vi "Online_Program_redesign_For_TV.vi"() -> ()   [LabVIEW 2014]
uses:
  <vilib>/Utility/file.llb/Read From Spreadsheet File (DBL).vi
  <vilib>/Analysis/Matrix/Numeric/Conversions/Array To Matrix - RA2.vi
  <vilib>/Instr/_visa.llb/VISA Configure Serial Port (Instr).vi
  <vilib>/Analysis/Matrix/Numeric/Conversions/Array To Matrix - RA.vi
  <vilib>/Utility/file.llb/Write To Spreadsheet File (DBL).vi
  <vilib>/Utility/file.llb/Write To Spreadsheet File (I64).vi
  <vilib>/Analysis/Matrix/NI_Matrix.lvlib
  NeuroSky_Dll_Call/Debug/NeuroSky_Dll_Call.dll
  user32.dll
panel:
  out "에러 출력":errorcluster
  out "메시지 2":string
  out "큐사인":bool
  out "icon_온도":bool
  out "icon_용변":bool
  out "icon_자판":bool
  out "icon_응급":bool=TRUE
  out "icon_기계":bool
  out "icon_침대":bool
  out "메시지":string
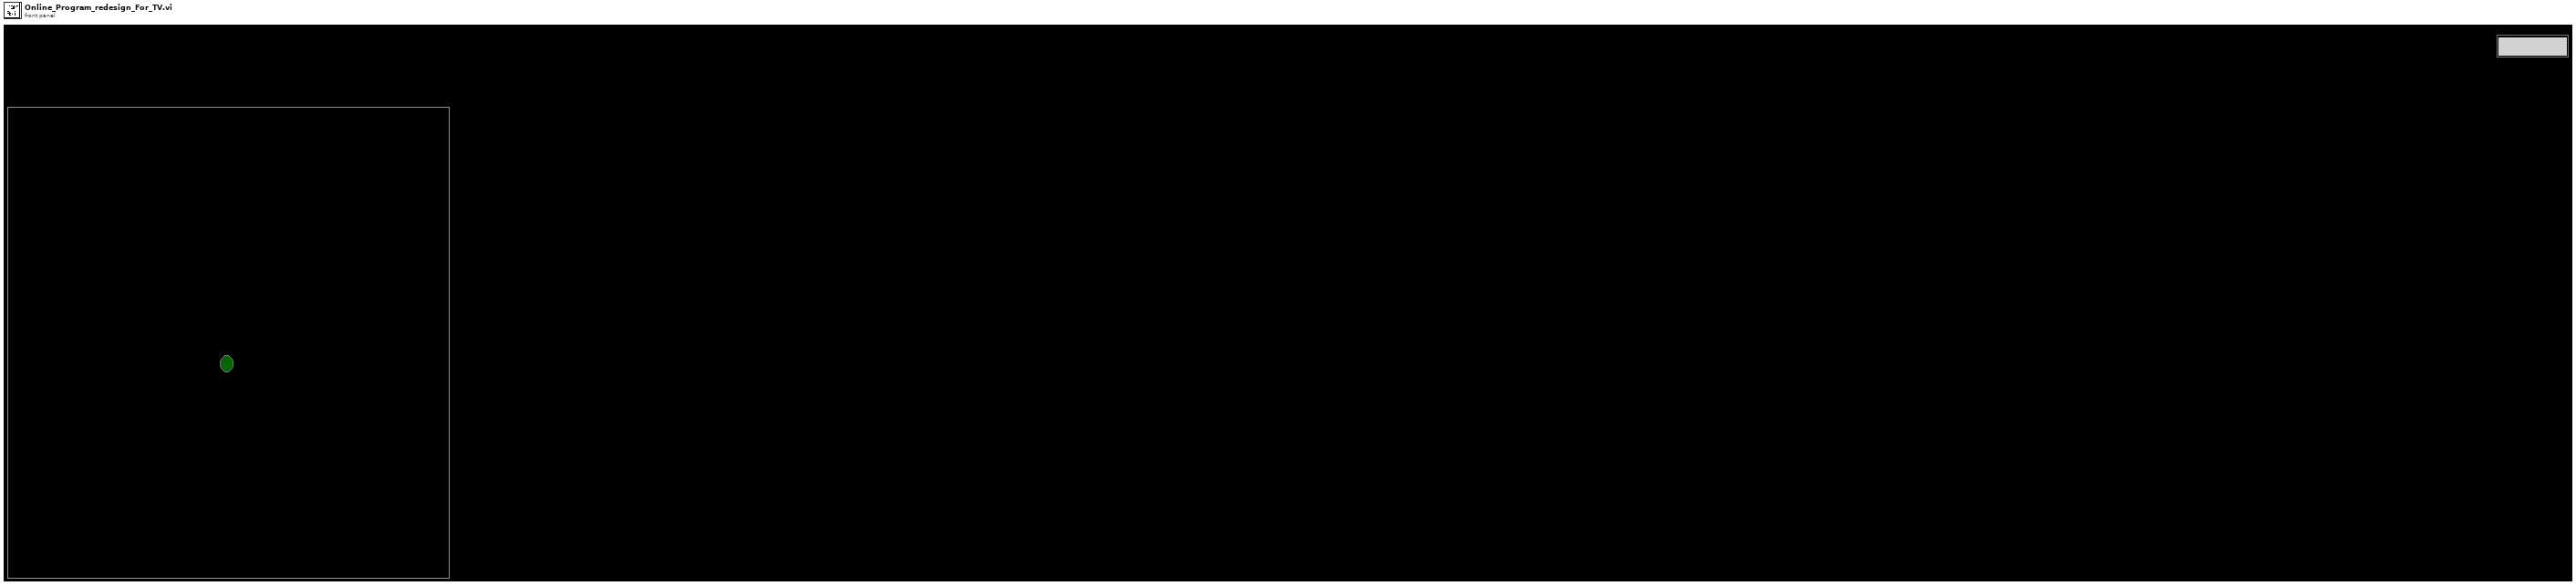
[diagram p1: front panel]
types:
  T1 = typedef "NI_Matrix.lvlib/RealMatrix.ctl" = dbl[][]
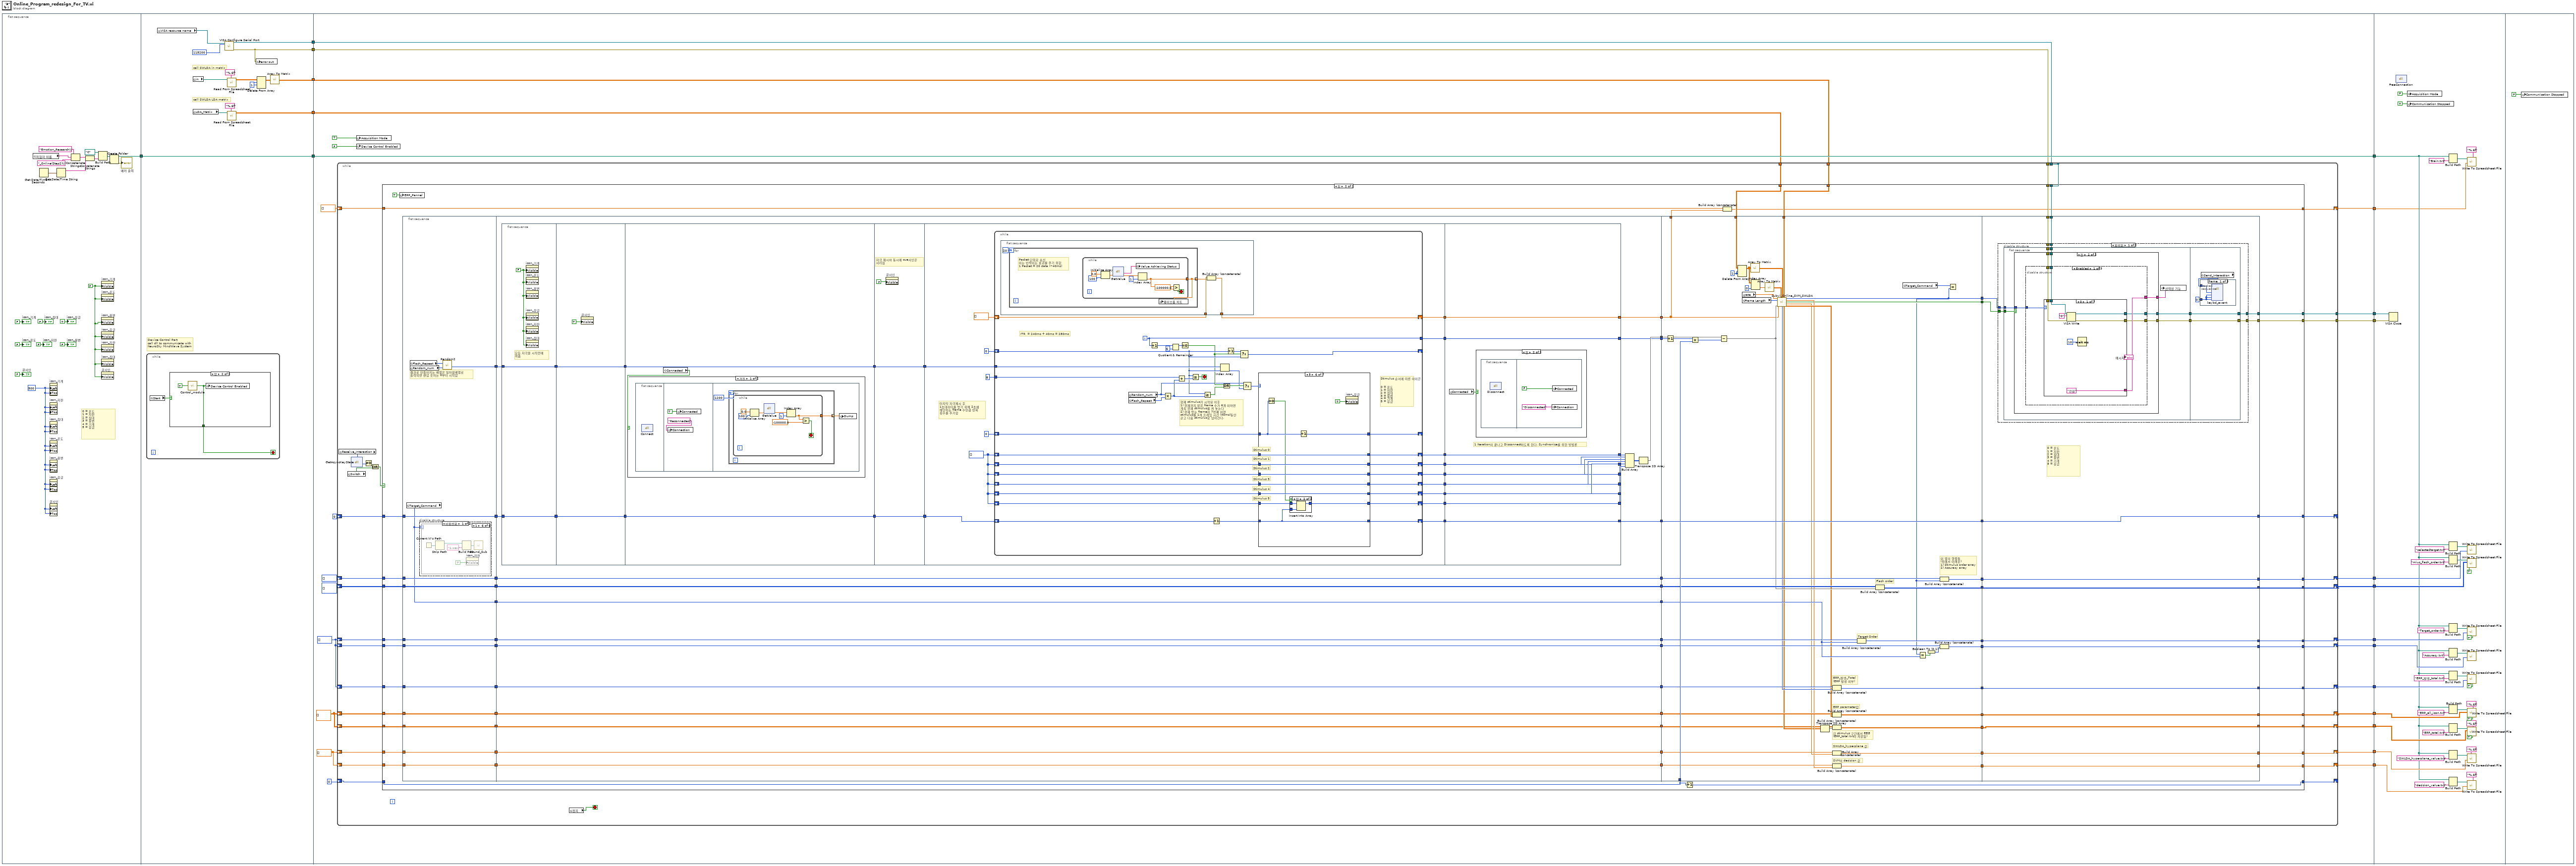
[diagram p0: block diagram]
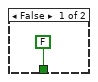
[diagram p2: hidden frame]
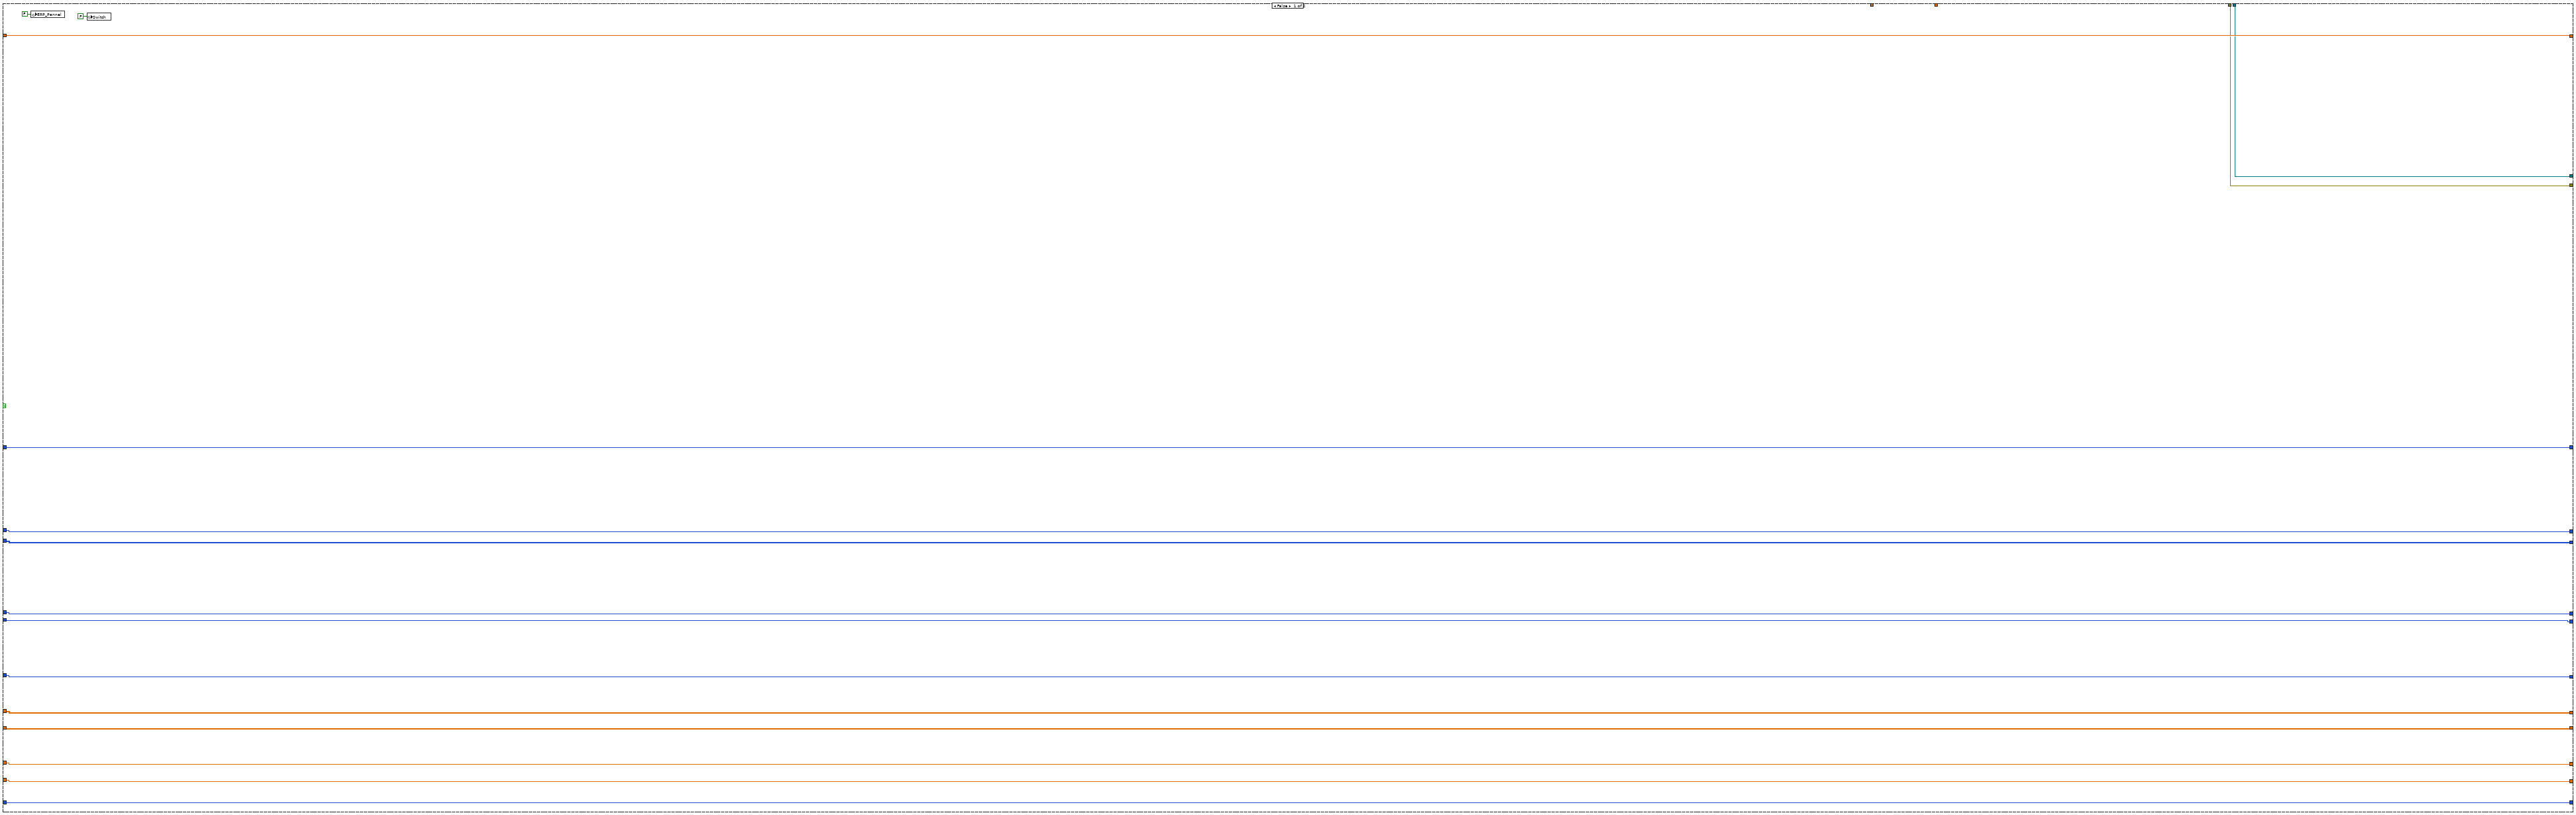
[diagram p3: hidden frame]
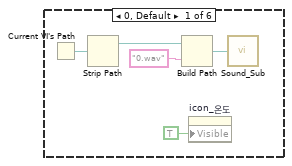
[diagram p4: hidden frame]
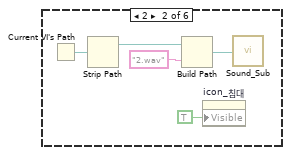
[diagram p5: hidden frame]
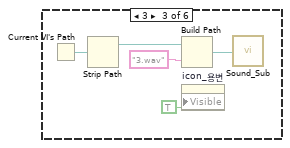
[diagram p6: hidden frame]
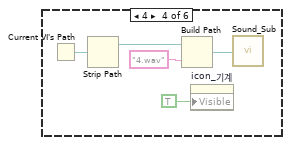
[diagram p7: hidden frame]
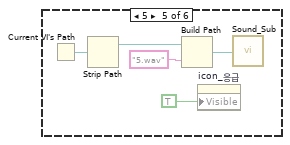
[diagram p8: hidden frame]
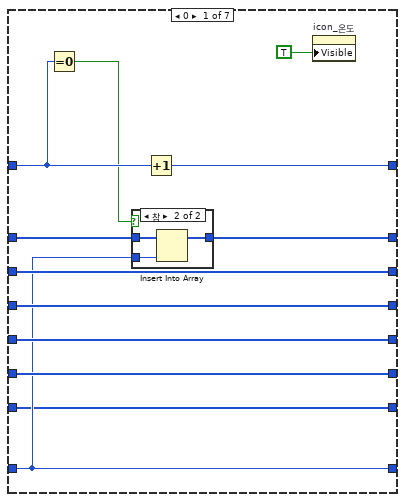
[diagram p11: hidden frame]
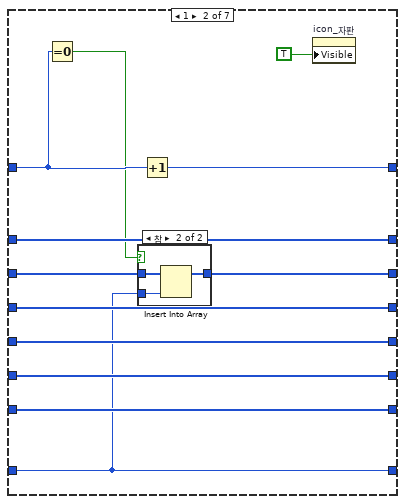
[diagram p13: hidden frame]
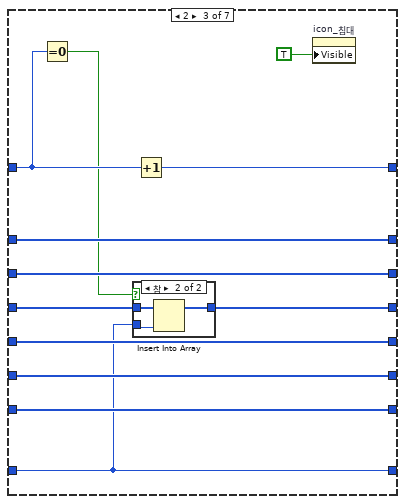
[diagram p15: hidden frame]
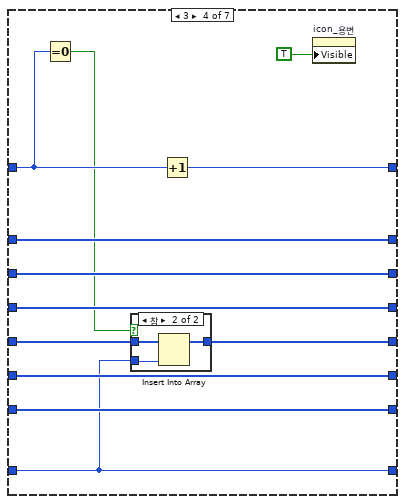
[diagram p17: hidden frame]
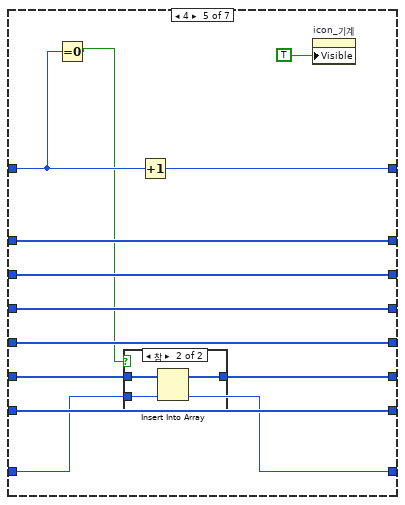
[diagram p19: hidden frame]
diagram:
  n1 = flat-sequence {
    tunnel: [w39] -> w19
    tunnel: w19 -> [w53]
    tunnel: [w53] -> w18
    tunnel: [w51] -> w17
    tunnel: [w44] -> w7
    tunnel: [w43] -> w4
    tunnel: [w40] -> w3
    tunnel: w18 -> [w76]
    tunnel: [w76] -> w16
    tunnel: [w85] -> w15
    tunnel: [w83] -> w14
    tunnel: [w81] -> w13
    tunnel: w17 -> [w65]
    tunnel: [w80] -> w12
    tunnel: [w77] -> w11
    tunnel: [w73] -> w10
    tunnel: [w71] -> w9
    tunnel: [w70] -> w8
    tunnel: w7 -> [w64]
    tunnel: [w68] -> w6
    tunnel: [w66] -> w5
    tunnel: w4 -> [w63]
    tunnel: w3 -> [w62]
    tunnel: [w61] -> w2
    tunnel: [w60] -> w1
    tunnel: w16 -> [w723]
    tunnel: w15 -> [w718]
    tunnel: w14 -> [w757]
    tunnel: w13 -> [w753]
    tunnel: w12 -> [w750]
    tunnel: w11 -> [w746]
    tunnel: w10 -> [w740]
    tunnel: w9 -> [w735]
    tunnel: w8 -> [w732]
    tunnel: w6 -> [w729]
    tunnel: w5 -> [w724]
    tunnel: w2 -> [w720]
    tunnel: w1 -> [w719]
    frame #0 {
      w20 = FALSE ("Visible")
      w22 = 500 ("Position:Left")
      # "0 = 온도\n1 = 자판\n2 = 침대\n3 = 용변 \n4 = 기계 \n5 = 응급"
      n2 = global read "Control_Panel_정리.vi" "피험자 이름"() -> (w30:string)
      n3 = Get Date/Time In Seconds() -> (seconds since 1Jan1904=w36:timestamp)
      n4 = property on="icon_기계" class="Bool (엄격한)"("Left"=w22, "Top"=w22) -> ()  [unwired: 2 in, 2 out]
      n5 = property on="icon_자판" class="Bool (엄격한)"("Left"=w22, "Top"=w22) -> ()  [unwired: 2 in, 2 out]
      n6 = property on="icon_침대" class="Bool (엄격한)"("Left"=w22, "Top"=w22) -> ()  [unwired: 2 in, 2 out]
      n7 = property on="icon_온도" class="Bool (엄격한)"("Left"=w22, "Top"=w22) -> ()  [unwired: 2 in, 2 out]
      n8 = property on="icon_용변" class="Bool (엄격한)"("Left"=w22, "Top"=w22) -> ()  [unwired: 2 in, 2 out]
      n9 = property on="icon_응급" class="Bool (엄격한)"("Left"=w22, "Top"=w22) -> ()  [unwired: 2 in, 2 out]
      n10 = property on="큐사인" class="Bool (엄격한)"("Left"=w22, "Top"=w22) -> ()  [unwired: 2 in, 2 out]
      n11 = Get Date/Time String(seconds (now)=w36) -> (date string=w37:string)  [unwired: 2 in, 1 out]
      n12 = Concatenate Strings("Emotion_Research\\" ("string"), w30, "_Online(Step2)\\" ("문자열")) -> (w32:string)
      n13 = Concatenate Strings(w32, w37) -> (w34:string)
      n14 = Build Path(base path=path "C:/" ("path"), name or relative path=w34) -> (appended path=w35:path)
      n15 = property on="icon_기계" class="Bool (엄격한)"("Visible"=w20) -> ()  [unwired: 2 in, 2 out]
      n16 = property on="icon_온도" class="Bool (엄격한)"("Visible"=w20) -> ()  [unwired: 2 in, 2 out]
      n17 = property on="icon_용변" class="Bool (엄격한)"("Visible"=w20) -> ()  [unwired: 2 in, 2 out]
      n18 = property on="icon_응급" class="Bool (엄격한)"("Visible"=w20) -> ()  [unwired: 2 in, 2 out]
      n19 = property on="icon_자판" class="Bool (엄격한)"("Visible"=w20) -> ()  [unwired: 2 in, 2 out]
      n20 = property on="icon_침대" class="Bool (엄격한)"("Visible"=w20) -> ()  [unwired: 2 in, 2 out]
      n21 = property on="큐사인" class="Bool (엄격한)"("Visible"=w20) -> ()  [unwired: 2 in, 2 out]
      n22 = Create Folder(path (use dialog)=w35) -> (created path=w39:path, error out=→"에러 출력":errorcluster)  [unwired: 2 in, 1 out]
      "icon_온도" <- FALSE ("icon_전원 6")
      "icon_용변" <- FALSE ("icon_전체종료")
      "icon_자판" <- FALSE ("icon_음량업 2")
      "icon_응급" <- TRUE ("icon_채널다운")
      "icon_기계" <- FALSE ("icon_음량다")
      "icon_침대" <- FALSE ("icon_채널업")
      "큐사인" <- FALSE ("icon_전원 7")
    }
    frame #1 {
      w47 = 1 ("인덱스 (행)")
      # "call SWLDA in matrix"
      # "call SWLDA LDA matrix"
      # "Device Control Part\ncall dll to communicate with\nNeuroSky MindWave System"
      n23 = while {
        stop <- w55 stop-if-true
        n24 = global read "Control_Panel_정리.vi" "Start"() -> (w54:bool)
        n25 = case shown="참" w54 {
          tunnel: [FALSE ("Connected") w57] -> w55
          frame False {
          }
          frame True {
            n26 = call "Control_module.vi"("Turn on"=TRUE ("Device Control Enabled")) -> ("Connected"=w57:bool)
            n27 = global write "Control_Panel_정리.vi" "Device Control Enabled"(w57) -> ()
          }
        }
      }
      n28 = global read "Control_Panel_정리.vi" "VISA resource name"() -> (w41:refnum<visa-resource-name>)
      n29 = global read "Control_Panel_정리.vi" "in"() -> (w45:path)
      n30 = global read "Control_Panel_정리.vi" "LDA_Matrix"() -> (w50:path)
      n31 = call-poly "VISA Configure Serial Port"("VISA resource name"=w41, "baud rate (9600)"=u32 115200) -> ("VISA resource name out"=w43:refnum<visa-resource-name>, "error out"=w40:errorcluster)  [unwired: 12 in]
      n32 = call-poly <vilib>:"Read From Spreadsheet File.vi"("format (%.3f)"="%.6f", "file path (dialog if empty)"=w45) -> ("all rows"=w46:dbl[][])  [unwired: 5 in, 4 out]
      n33 = call-poly <vilib>:"Read From Spreadsheet File.vi"("format (%.3f)"="%.6f", "file path (dialog if empty)"=w50) -> ("all rows"=w51:dbl[][])  [unwired: 5 in, 4 out]
      n34 = global write "Control_Panel_정리.vi" "error out"(w40) -> ()
      n35 = Delete From Array(array=w46, length=w47, index (row)=w47) -> (array with subset deleted=w48:dbl[][])  [unwired: 1 in, 1 out]
      n36 = call-poly <vilib>:"Array To Matrix.vi"("Real 2D Array"=w48) -> ("Real Matrix"=w44:T1)
    }
    frame #2 {
      w69 = dbl[] []
      w67 = dbl[][] []
      w72 = i16[] []
      n37 = while {
        shift-right: [w94] -> w85
        shift-left: dbl[] [] -> [w100]
        shift-right: [w120] -> _
        shift-left: 0 ("y") -> [w121]
        shift-right: [w114] -> w83
        shift-left: i32[][] [] -> [w115]
        shift-right: [w118] -> w81
        shift-left: i32[] [] -> [w119]
        shift-right: [w116] -> w80
        shift-left: w72 -> [w117]
        shift-right: [w112] -> w77
        shift-left: w72 -> [w113]
        shift-right: [w111] -> w73
        shift-left: w72 -> [w110]
        shift-right: [w109] -> w71
        shift-left: w67 -> [w108]
        shift-right: [w107] -> w70
        shift-left: w69 -> [w106]
        shift-right: [w105] -> w68
        shift-left: w69 -> [w104]
        shift-right: [w103] -> w66
        shift-left: w67 -> [w102]
        tunnel: w65 -> [w101]
        tunnel: w64 -> [w99]
        tunnel: [w97] -> _
        tunnel: w63 -> [w97]
        tunnel: w62 -> [w98]
        tunnel: [w96] -> w61
        tunnel: [w95] -> w60
        shift-right: [w86] -> _
        shift-left: 0 -> [w87]
        stop <- w88 stop-if-true
        n38 = global read "Control_Panel_정리.vi" "Receive_Interaction"() -> (w92:u8)
        n39 = global read "Control_Panel_정리.vi" "Switch"() -> (w91:bool)
        n40 = dll-call lib="User32.dll" fn="GetAsyncKeyState"("vKey"=w92) -> ("return type"=w93:i64)  [unwired: 4 in, 2 out]
        n41 = Not Equal To 0?(x=w93) -> (x != 0?=w90:bool)
        n42 = Or(x=w90, y=w91) -> (x .or. y?=w89:bool)
        n43 = case shown="참" w89 {
          tunnel: w121 -> [w132 w169]
          tunnel: [w132 w168] -> w120
          tunnel: w119 -> [w131 w167]
          tunnel: [w131 w166] -> w118
          tunnel: w117 -> [w128 w165]
          tunnel: [w128 w164] -> w116
          tunnel: w115 -> [w130 w163]
          tunnel: [w130 w162] -> w114
          tunnel: w113 -> [w129 w161]
          tunnel: [w129 w160] -> w112
          tunnel: [w127 w159] -> w111
          tunnel: w110 -> [w127 w158]
          tunnel: [w126 w157] -> w109
          tunnel: w108 -> [w126 w156]
          tunnel: [w124 w155] -> w107
          tunnel: w106 -> [w124 w154]
          tunnel: [w123 w153] -> w105
          tunnel: w104 -> [w123 w152]
          tunnel: [w125 w151] -> w103
          tunnel: w102 -> [w125 w150]
          tunnel: w101 -> [_ w149]
          tunnel: w100 -> [w135 w148]
          tunnel: w99 -> [_ w146]
          tunnel: w98 -> [w133 w145]
          tunnel: w97 -> [w134 w144]
          tunnel: [w134 w143] -> w96
          tunnel: [w133 w142] -> w95
          tunnel: [w135 w141] -> w94
          tunnel: w87 -> [w122 w139]
          tunnel: [w122 w138] -> w86
          frame False {
            n44 = global write "Control_Panel_정리.vi" "ERP_Pannel"(FALSE ("ERP_Pannel")) -> ()
            n45 = global write "Control_Panel_정리.vi" "Switch"(FALSE ("Switch")) -> ()
          }
          frame True {
            n46 = global write "Control_Panel_정리.vi" "ERP_Pannel"(TRUE ("ERP_Pannel")) -> ()
            n47 = flat-sequence {
              tunnel: [w221] -> w207
              tunnel: w169 -> [w220]
              tunnel: [w220] -> w206
              tunnel: [w208] -> w205
              tunnel: w167 -> [w217]
              tunnel: [w217] -> w204
              tunnel: w165 -> [w216]
              tunnel: [w216] -> w203
              tunnel: w163 -> [w215]
              tunnel: [w215] -> w202
              tunnel: [w214] -> w201
              tunnel: w161 -> [w214]
              tunnel: w158 -> [w213]
              tunnel: [w213] -> w200
              tunnel: w156 -> [w212]
              tunnel: [w212] -> w199
              tunnel: w154 -> [w211]
              tunnel: [w211] -> w198
              tunnel: w152 -> [w210]
              tunnel: [w210] -> w197
              tunnel: w150 -> [w209]
              tunnel: [w209] -> w196
              tunnel: w207 -> [w292]
              tunnel: w206 -> [w289]
              tunnel: [w290] -> w195
              tunnel: [w279] -> w194
              tunnel: [w288] -> w193
              tunnel: [w287] -> w192
              tunnel: w205 -> [w286]
              tunnel: [w286] -> w191
              tunnel: w204 -> [w285]
              tunnel: [w285] -> w190
              tunnel: [w284] -> w189
              tunnel: w203 -> [w284]
              tunnel: [w283] -> w188
              tunnel: w202 -> [w283]
              tunnel: [w282] -> w187
              tunnel: w201 -> [w282]
              tunnel: [w281] -> w186
              tunnel: w200 -> [w281]
              tunnel: [w280] -> w185
              tunnel: w199 -> [w280]
              tunnel: [w278] -> w184
              tunnel: w198 -> [w278]
              tunnel: [w277] -> w183
              tunnel: w197 -> [w277]
              tunnel: w196 -> [w276]
              tunnel: [w276] -> w182
              tunnel: w195 -> [w533]
              tunnel: w194 -> [w507]
              tunnel: w193 -> [w546]
              tunnel: w192 -> [w547]
              tunnel: w139 -> [w545]
              tunnel: [w546] -> w171
              tunnel: [w505] -> w172
              tunnel: w191 -> [w532]
              tunnel: w190 -> [w541]
              tunnel: [w540] -> w173
              tunnel: w189 -> [w538]
              tunnel: [w537] -> w174
              tunnel: w188 -> [w536]
              tunnel: [w534] -> w175
              tunnel: w187 -> [w531]
              tunnel: [w530] -> w176
              tunnel: [w528] -> w177
              tunnel: w186 -> [w527]
              tunnel: [w525] -> w178
              tunnel: w185 -> [w524]
              tunnel: [w522] -> w179
              tunnel: w184 -> [w521]
              tunnel: [w519] -> w180
              tunnel: w183 -> [w518]
              tunnel: [w515] -> w181
              tunnel: w182 -> [w514]
              tunnel: w149 -> [w513]
              tunnel: [w507] -> w147
              tunnel: w146 -> [w509]
              tunnel: [w508] -> w170
              tunnel: [w568] -> w168
              tunnel: [w567] -> w166
              tunnel: [w564] -> w164
              tunnel: [w566] -> w162
              tunnel: [w565] -> w160
              tunnel: [w563] -> w159
              tunnel: [w562] -> w157
              tunnel: [w561] -> w155
              tunnel: [w560] -> w153
              tunnel: [w559] -> w151
              tunnel: w181 -> [w559]
              tunnel: w180 -> [w560]
              tunnel: w179 -> [w561]
              tunnel: w178 -> [w562]
              tunnel: w177 -> [w563]
              tunnel: w176 -> [w565]
              tunnel: w175 -> [w566]
              tunnel: w174 -> [w564]
              tunnel: w173 -> [w567]
              tunnel: w172 -> [w558]
              tunnel: w171 -> [w568]
              tunnel: w170 -> [w557]
              tunnel: w145 -> [w556]
              tunnel: w144 -> [w555]
              tunnel: [w554] -> w143
              tunnel: [w553] -> w142
              frame #0 {
                # "결과로 만들어지는 배열은 일차원배열로\n출력되면 랜덤 숫자는 0부터 시작함"
                n48 = global read "Control_Panel_정리.vi" "Target_Command"() -> (w208:i32)
                n49 = global read "Control_Panel_정리.vi" "Flash_Repeat"() -> (w219:i32)
                n50 = global read "Control_Panel_정리.vi" "Random_num"() -> (w218:i32)
                n51 = disable-structure shown="비활성화" {
                  disable-tunnel: w208 -> [w222 _]
                  frame Disabled {
                    n52 = case shown="1" w222 {
                      frame 0, Default {
                        n53 = Current VI's Path() -> (path=w225:path)
                        n54 = Strip Path(path=w225) -> (stripped path=w226:path)  [unwired: 1 out]
                        n55 = Build Path(base path=w226, name or relative path="0.wav" ("이름 또는 상대 경로")) -> (appended path=w224:path)
                        n56 = property on="icon_온도" class="Bool (엄격한)"("Visible"=TRUE) -> ()  [unwired: 2 in, 2 out]
                        n57 = call "Sound_Sub.vi"("path"=w224) -> ()
                      }
                      frame 2 {
                        n58 = Current VI's Path() -> (path=w229:path)
                        n59 = Strip Path(path=w229) -> (stripped path=w230:path)  [unwired: 1 out]
                        n60 = Build Path(base path=w230, name or relative path="2.wav" ("이름 또는 상대 경로")) -> (appended path=w232:path)
                        n61 = property on="icon_침대" class="Bool (엄격한)"("Visible"=TRUE) -> ()  [unwired: 2 in, 2 out]
                        n62 = call "Sound_Sub.vi"("path"=w232) -> ()
                      }
                      frame 3 {
                        n63 = Current VI's Path() -> (path=w234:path)
                        n64 = Strip Path(path=w234) -> (stripped path=w235:path)  [unwired: 1 out]
                        n65 = Build Path(base path=w235, name or relative path="3.wav" ("이름 또는 상대 경로")) -> (appended path=w237:path)
                        n66 = property on="icon_용변" class="Bool (엄격한)"("Visible"=TRUE) -> ()  [unwired: 2 in, 2 out]
                        n67 = call "Sound_Sub.vi"("path"=w237) -> ()
                      }
                      frame 4 {
                        n68 = Current VI's Path() -> (path=w239:path)
                        n69 = Strip Path(path=w239) -> (stripped path=w240:path)  [unwired: 1 out]
                        n70 = Build Path(base path=w240, name or relative path="4.wav" ("이름 또는 상대 경로")) -> (appended path=w242:path)
                        n71 = property on="icon_기계" class="Bool (엄격한)"("Visible"=TRUE) -> ()  [unwired: 2 in, 2 out]
                        n72 = call "Sound_Sub.vi"("path"=w242) -> ()
                      }
                      frame 5 {
                        n73 = Current VI's Path() -> (path=w244:path)
                        n74 = Strip Path(path=w244) -> (stripped path=w245:path)  [unwired: 1 out]
                        n75 = Build Path(base path=w245, name or relative path="5.wav" ("이름 또는 상대 경로")) -> (appended path=w247:path)
                        n76 = property on="icon_응급" class="Bool (엄격한)"("Visible"=TRUE) -> ()  [unwired: 2 in, 2 out]
                        n77 = call "Sound_Sub.vi"("path"=w247) -> ()
                      }
                      frame 1 {
                        n78 = Current VI's Path() -> (path=w250:path)
                        n79 = Strip Path(path=w250) -> (stripped path=w251:path)  [unwired: 1 out]
                        n80 = Build Path(base path=w251, name or relative path="1.wav" ("이름 또는 상대 경로")) -> (appended path=w249:path)
                        n81 = property on="icon_자판" class="Bool (엄격한)"("Visible"=TRUE) -> ()  [unwired: 2 in, 2 out]
                        n82 = call "Sound_Sub.vi"("path"=w249) -> ()
                      }
                    }
                  }
                  frame Enabled {
                  }
                }
                n83 = call "Random2.vi"("Random_num"=w218, "전체횟수"=w219) -> ("배열"=w221:i32[])
              }
              frame #1 {
                n84 = flat-sequence {
                  tunnel: w289 -> [w294]
                  tunnel: w292 -> [w295]
                  tunnel: [w295] -> w275
                  tunnel: [w294] -> w274
                  tunnel: [w298] -> w267
                  tunnel: [w297] -> w266
                  tunnel: w275 -> [w298]
                  tunnel: w274 -> [w297]
                  tunnel: w267 -> [w301]
                  tunnel: [w301] -> w256
                  tunnel: w266 -> [w300]
                  tunnel: [w300] -> w254
                  tunnel: w256 -> [w317]
                  tunnel: [w317] -> w255
                  tunnel: w254 -> [w316]
                  tunnel: [w316] -> w253
                  tunnel: w255 -> [w333]
                  tunnel: w253 -> [w323]
                  tunnel: [w331] -> w265
                  tunnel: [w330] -> w264
                  tunnel: [w329] -> w263
                  tunnel: [w328] -> w262
                  tunnel: [w327] -> w261
                  tunnel: [w322] -> w260
                  tunnel: [w321] -> w259
                  tunnel: [w320] -> w258
                  tunnel: [w318] -> w257
                  tunnel: [w494] -> w279
                  tunnel: [w495] -> w270
                  tunnel: [w496] -> w287
                  tunnel: [w497] -> w288
                  tunnel: [w498] -> w273
                  tunnel: [w499] -> w272
                  tunnel: [w500] -> w271
                  tunnel: [w501] -> w269
                  tunnel: [w502] -> w268
                  tunnel: w265 -> [w502]
                  tunnel: w264 -> [w501]
                  tunnel: w263 -> [w500]
                  tunnel: w262 -> [w499]
                  tunnel: w261 -> [w498]
                  tunnel: w260 -> [w497]
                  tunnel: w259 -> [w496]
                  tunnel: w258 -> [w495]
                  tunnel: w257 -> [w494]
                  frame #0 {
                    w293 = FALSE ("Visible")
                    # "모든 자극을 시작전에\n꺼줌"
                    n85 = property on="icon_기계" class="Bool (엄격한)"("Visible"=w293) -> ()  [unwired: 2 in, 2 out]
                    n86 = property on="icon_온도" class="Bool (엄격한)"("Visible"=w293) -> ()  [unwired: 2 in, 2 out]
                    n87 = property on="icon_용변" class="Bool (엄격한)"("Visible"=w293) -> ()  [unwired: 2 in, 2 out]
                    n88 = property on="icon_응급" class="Bool (엄격한)"("Visible"=w293) -> ()  [unwired: 2 in, 2 out]
                    n89 = property on="icon_자판" class="Bool (엄격한)"("Visible"=w293) -> ()  [unwired: 2 in, 2 out]
                    n90 = property on="icon_침대" class="Bool (엄격한)"("Visible"=w293) -> ()  [unwired: 2 in, 2 out]
                  }
                  frame #1 {
                    n91 = property on="큐사인" class="Bool (엄격한)"("Visible"=TRUE) -> ()  [unwired: 2 in, 2 out]
                  }
                  frame #2 {
                    n92 = global read "Control_Panel_정리.vi" "Connected"() -> (w299:bool)
                    n93 = case shown="거짓" w299 {
                      frame False {
                        n94 = flat-sequence {
                          frame #0 {
                            n95 = dll-call lib="C:/Users/Server/Desktop/NeuroSky/NeuroSky_Dll_Call/Debug/NeuroSky_Dll_Call.dll" fn="Connect"() -> ()  [unwired: 4 in, 2 out]
                          }
                          frame #1 {
                            n96 = global write "Control_Panel_정리.vi" "Connection"("Reconnected") -> ()
                            n97 = global write "Control_Panel_정리.vi" "Connected"(TRUE ("Connected")) -> ()
                          }
                          frame #2 {
                            n98 = for {
                              N: 1200 -> [_]
                              tunnel: [w306] -> w304 mode=indexing
                              n99 = while {
                                tunnel: [w308] -> w306
                                stop <- w307 stop-if-true
                                n100 = Initialize Array(0.0 ("element"), 100 ("dimension size")) -> (w313:dbl[])
                                n101 = dll-call lib="C:/Users/Server/Desktop/NeuroSky/NeuroSky_Dll_Call/Debug/NeuroSky_Dll_Call.dll" fn="GetValue"("result"=w313) -> ("result"=w314:dbl[])  [unwired: 4 in, 2 out]
                                n102 = Index Array(array=w314, index=1) -> (element=w308:dbl)
                                n103 = Greater?(x=w308, y=-100000.0) -> (0:w307:bool)
                              }
                            }
                            n104 = global write "Control_Panel_정리.vi" "Dump"(w304) -> ()
                          }
                        }
                      }
                      frame True {
                      }
                    }
                  }
                  frame #3 {
                    # "자극 제시와 동시에 cue사인은\n사라짐"
                    n105 = property on="큐사인" class="Bool (엄격한)"("Visible"=FALSE) -> ()  [unwired: 2 in, 2 out]
                  }
                  frame #4 {
                    w325 = i32[] []
                    # "마지막 자극제시 후\n1초데이터를 받기 위해 2초에\n해당하는 frame 수만큼 반복\n횟수를 추가함"
                    n106 = while {
                      tunnel: w333 -> [w369]
                      shift-right: [w337] -> w318
                      shift-left: dbl[] [] -> [w338]
                      tunnel: 8 -> [w334]
                      shift-right: [w366] -> w331
                      shift-left: w325 -> [w365]
                      shift-right: [w363] -> w330
                      shift-left: w325 -> [w364]
                      shift-right: [w361] -> w320
                      shift-left: w325 -> [w362]
                      shift-right: [w359] -> w329
                      shift-left: w325 -> [w360]
                      shift-right: [w357] -> w328
                      shift-left: w325 -> [w358]
                      shift-right: [w356] -> w327
                      shift-left: w325 -> [w343]
                      shift-right: [w354] -> w322
                      shift-left: w323 -> [w355]
                      shift-right: [w350] -> _
                      shift-left: 0 -> [w349]
                      shift-right: [w344] -> _
                      shift-left: 0 ("y") -> [w345]
                      tunnel: [w339] -> w321
                      i -> [w339]
                      stop <- w370 stop-if-true
                      # "ITR  = 240ms + 40ms = 280ms"
                      # "현재 stimulus가 시작된 이후\n1) 현재까지 받은 frame 수가 6개 이하면\n계속 현재 stimulus를 켜 놓는다\n2) 현재 받는 frame이 7번째 이면\nstimulus를 1개 프레임 시간 (40ms)동안\n끈고 다음 stimulus로 넘어간다."
                      # "Stimulus 순서에 따른 아이콘\n\n\n0 = 온도\n1 = 자판\n2 = 침대\n3 = 용변 \n4 = 기계 \n5 = 응급"
                      # "Stimulus 5"
                      # "Stimulus 4"
                      # "Stimulus 3"
                      # "Stimulus 2"
                      # "Stimulus 1"
                      # "Stimulus 0"
                      n107 = flat-sequence {
                        tunnel: [w375] -> w337
                        tunnel: w338 -> [w374]
                        frame #0 {
                          n108 = for {
                            N: 20 -> [_]
                            tunnel: [w376] -> w373 mode=indexing
                            # "Packet 단위로 송신\n이는 반짝이는 효과를 주기 위함\n1 Packet = 20 data (~40ms)"
                            n109 = while {
                              tunnel: [w378] -> w376
                              stop <- w377 stop-if-true
                              n110 = Initialize Array(0.0 ("element"), 100 ("dimension size")) -> (w384:dbl[])
                              n111 = dll-call lib="C:/Users/Server/Desktop/NeuroSky/NeuroSky_Dll_Call/Debug/NeuroSky_Dll_Call.dll" fn="GetValue"("result"=w384) -> ("errCode"=w380:string, "result"=w385:dbl[])  [unwired: 3 in, 2 out]
                              n112 = global write "Control_Panel_정리.vi" "Value Achieving Status"(w380) -> ()
                              n113 = Index Array(array=w385, index=1) -> (element=w378:dbl)
                              n114 = Greater?(x=w378, y=-100000.0) -> (0:w377:bool)
                            }
                            n115 = global write "Control_Panel_정리.vi" "웨이브폼 차트"(w376) -> ()
                          }
                          n116 = Build Array (concatenate)(w374, w373) -> (w375:dbl[])
                        }
                      }
                      n117 = global read "Control_Panel_정리.vi" "Random_num"() -> (w336:i32)
                      n118 = global read "Control_Panel_정리.vi" "Flash_Repeat"() -> (w335:i32)
                      n119 = Increment(x=w339) -> (x+1=w342:i32)
                      n120 = Multiply(x=w336, y=w335) -> (x*y=w340:i32)
                      n121 = Quotient & Remainder(x=w342, y=6) -> (x-y*floor(x/y)=w352:i32)  [unwired: 1 out]
                      n122 = Add(x=w334, y=w340) -> (x+y=w371:i32)
                      n123 = Equal To 0?(x=w352) -> (x = 0?=w348:bool)
                      n124 = Greater Or Equal?(x=w349, y=w371) -> (x >= y?=w370:bool)
                      n125 = Greater Or Equal?(x=w349, y=w340) -> (x >= y?=w347:bool)
                      n126 = Increment(x=w355) -> (x+1=w367:i32)
                      n127 = Index Array(array=w369, index=w349) -> (element=w341:i32)
                      n128 = Or(x=w348, y=w347) -> (x .or. y?=w346:bool)
                      n129 = Increment(x=w349) -> (x+1=w351:i32)
                      n130 = Select(t=w351, s=w348, f=w349) -> (s? t:f=w350:i32)
                      n131 = Select(t=w336, s=w346, f=w341) -> (s? t:f=w368:i32)
                      n132 = case shown="5" w368 {
                        tunnel: w367 -> [w391 w407 w422 w438 w454 w471 w486]
                        tunnel: [w396 w404 w429 w445 w461 w477 w492] -> w366
                        tunnel: w365 -> [w397 w404 w429 w445 w461 w477 w492]
                        tunnel: w364 -> [w395 w413 w426 w442 w458 w475 w491]
                        tunnel: [w395 w412 w426 w442 w458 w475 w491] -> w363
                        tunnel: w362 -> [w394 w411 w428 w441 w457 w474 w490]
                        tunnel: [w394 w411 w427 w441 w457 w474 w490] -> w361
                        tunnel: w360 -> [w393 w410 w425 w444 w456 w473 w489]
                        tunnel: [w393 w410 w425 w443 w456 w473 w489] -> w359
                        tunnel: w358 -> [w392 w409 w424 w440 w460 w472 w488]
                        tunnel: [w392 w409 w424 w440 w459 w472 w488] -> w357
                        tunnel: w343 -> [w388 w408 w423 w439 w455 w476 w487]
                        tunnel: [w388 w408 w423 w439 w455 w468 w487] -> w356
                        tunnel: [w391 w407 w422 w438 w454 w471 w486] -> w354
                        tunnel: w345 -> [w390 w406 w421 w436 w453 w469 _]
                        tunnel: [w389 w405 w420 w437 w452 w470 0] -> w344
                        frame 0 {
                          n133 = Equal To 0?(x=w390) -> (x = 0?=w386:bool)
                          n134 = case shown="참" w386 {
                            tunnel: w397 -> [w398 w401]
                            tunnel: [w398 w400] -> w396
                            tunnel: w391 -> [_ w399]
                            frame False {
                            }
                            frame True {
                              n135 = Insert Into Array(array=w401, new element=w399) -> (w400:i32[])  [unwired: 1 in]
                            }
                          }
                          n136 = Increment(x=w390) -> (x+1=w389:i32)
                          n137 = property on="icon_온도" class="Bool (엄격한)"("Visible"=TRUE) -> ()  [unwired: 2 in, 2 out]
                        }
                        frame 1 {
                          n138 = Equal To 0?(x=w406) -> (x = 0?=w402:bool)
                          n139 = case shown="참" w402 {
                            tunnel: w413 -> [w414 w417]
                            tunnel: [w414 w416] -> w412
                            tunnel: w407 -> [_ w415]
                            frame False {
                            }
                            frame True {
                              n140 = Insert Into Array(array=w417, new element=w415) -> (w416:i32[])  [unwired: 1 in]
                            }
                          }
                          n141 = Increment(x=w406) -> (x+1=w405:i32)
                          n142 = property on="icon_자판" class="Bool (엄격한)"("Visible"=TRUE) -> ()  [unwired: 2 in, 2 out]
                        }
                        frame 2 {
                          n143 = Equal To 0?(x=w421) -> (x = 0?=w418:bool)
                          n144 = case shown="참" w418 {
                            tunnel: w428 -> [w430 w433]
                            tunnel: [w430 w432] -> w427
                            tunnel: w422 -> [_ w431]
                            frame False {
                            }
                            frame True {
                              n145 = Insert Into Array(array=w433, new element=w431) -> (w432:i32[])  [unwired: 1 in]
                            }
                          }
                          n146 = Increment(x=w421) -> (x+1=w420:i32)
                          n147 = property on="icon_침대" class="Bool (엄격한)"("Visible"=TRUE) -> ()  [unwired: 2 in, 2 out]
                        }
                        frame 3 {
                          n148 = Equal To 0?(x=w436) -> (x = 0?=w434:bool)
                          n149 = case shown="참" w434 {
                            tunnel: w444 -> [w446 w449]
                            tunnel: [w446 w448] -> w443
                            tunnel: w438 -> [_ w447]
                            frame False {
                            }
                            frame True {
                              n150 = Insert Into Array(array=w449, new element=w447) -> (w448:i32[])  [unwired: 1 in]
                            }
                          }
                          n151 = Increment(x=w436) -> (x+1=w437:i32)
                          n152 = property on="icon_용변" class="Bool (엄격한)"("Visible"=TRUE) -> ()  [unwired: 2 in, 2 out]
                        }
                        frame 4 {
                          n153 = Equal To 0?(x=w453) -> (x = 0?=w450:bool)
                          n154 = case shown="참" w450 {
                            tunnel: w460 -> [w462 w465]
                            tunnel: [w462 w464] -> w459
                            tunnel: w454 -> [_ w463]
                            frame False {
                            }
                            frame True {
                              n155 = Insert Into Array(array=w465, new element=w463) -> (w464:i32[])  [unwired: 1 in]
                            }
                          }
                          n156 = Increment(x=w453) -> (x+1=w452:i32)
                          n157 = property on="icon_기계" class="Bool (엄격한)"("Visible"=TRUE) -> ()  [unwired: 2 in, 2 out]
                        }
                        frame 5 {
                          n158 = Equal To 0?(x=w469) -> (x = 0?=w466:bool)
                          n159 = case shown="참" w466 {
                            tunnel: w476 -> [w478 w481]
                            tunnel: [w478 w480] -> w468
                            tunnel: w471 -> [_ w479]
                            frame False {
                            }
                            frame True {
                              n160 = Insert Into Array(array=w481, new element=w479) -> (w480:i32[])  [unwired: 1 in]
                            }
                          }
                          n161 = Increment(x=w469) -> (x+1=w470:i32)
                          n162 = property on="icon_응급" class="Bool (엄격한)"("Visible"=TRUE) -> ()  [unwired: 2 in, 2 out]
                        }
                        frame 6, Default {
                          w483 = FALSE ("Visible")
                          w484 = FALSE ("Visible")
                          w482 = FALSE ("Visible")
                          n163 = property on="icon_기계" class="Bool (엄격한)"("Visible"=w482) -> ()  [unwired: 2 in, 2 out]
                          n164 = property on="icon_온도" class="Bool (엄격한)"("Visible"=w482) -> ()  [unwired: 2 in, 2 out]
                          n165 = property on="icon_응급" class="Bool (엄격한)"("Visible"=w484) -> ()  [unwired: 2 in, 2 out]
                          n166 = property on="icon_용변" class="Bool (엄격한)"("Visible"=w484) -> ()  [unwired: 2 in, 2 out]
                          n167 = property on="icon_자판" class="Bool (엄격한)"("Visible"=w483) -> ()  [unwired: 2 in, 2 out]
                          n168 = property on="icon_침대" class="Bool (엄격한)"("Visible"=w483) -> ()  [unwired: 2 in, 2 out]
                        }
                      }
                    }
                  }
                  frame #5 {
                    # "1 Iteration이 끝나고 Disconnect하도록 한다. Synchronize를 위한 방법론"
                    n169 = global read "Control_Panel_정리.vi" "Connected"() -> (w493:bool)
                    n170 = case shown="참" w493 {
                      frame False {
                      }
                      frame True {
                        n171 = flat-sequence {
                          frame #0 {
                            n172 = dll-call lib="C:/Users/Server/Desktop/NeuroSky/NeuroSky_Dll_Call/Debug/NeuroSky_Dll_Call.dll" fn="Disconnect"() -> ()  [unwired: 4 in, 2 out]
                          }
                          frame #1 {
                            n173 = global write "Control_Panel_정리.vi" "Connection"("Disconnected") -> ()
                            n174 = global write "Control_Panel_정리.vi" "Connected"(FALSE ("Connected")) -> ()
                          }
                        }
                      }
                    }
                  }
                }
                n175 = Build Array(w268, w269, w270, w271, w272, w273) -> (w291:i32[][])
                n176 = Transpose 2D Array(2D array=w291) -> (transposed array=w290:i32[][])
              }
              frame #2 {
                w550 = 1 ("인덱스 (행)")
                # "각 stimulus 구간에서 EEG\n(ERP_total.txt라 저장됨)"
                # "ERP parameter값"
                # "SVM의 decision 값"
                # "SWLDA_hyperplane 값"
                # "ERP_발생_Total\n(ERP 발생 여부)"
                # "Target Order"
                # "Flash order"
                # "이 열의 행렬들 \n(위에서 아래로)\n1) Stimulus order array\n2) Accuracy array"
                n177 = Increment(x=w547) -> (x+1=w551:i32)
                n178 = Multiply(x=w551, y=w545) -> (x*y=w552:i32)
                n179 = Subtract(x=w533, y=w552) -> (x-y=w535:i32[][])
                n180 = Delete From Array(array=w513, length=w550, index (row)=w550) -> (array with subset deleted=w511:dbl[][])  [unwired: 1 in, 1 out]
                n181 = global read "Control_Panel_정리.vi" "rate"() -> (w543:dbl)
                n182 = global read "Control_Panel_정리.vi" "Frame Length"() -> (w544:i32)
                n183 = call-poly <vilib>:"Array To Matrix.vi"("Real 2D Array"=w511) -> ("Real Matrix"=w510:T1)
                n184 = Index Array(array=w511, index (col)=0 ("인덱스")) -> (element=w512:dbl[])  [unwired: 1 in]
                n185 = call-poly <vilib>:"Array To Matrix.vi"("Real 1D Array"=w512) -> ("Real Matrix (Column Vector)"=w548:T1)
                n186 = call "Subvi_Online_SVM_SWLDA.vi"("rate"=w543, "Value"=w548, "Matrix"=w510, "in"=w509, "samples per channel"=w544, "Brain_data_source"=w507, "Target_Flash_Order"=w535) -> ("output-0~8"=w505:i32, "decision"=w520:dbl[], "ERP_발생여부"=w508:bool, "SWLDA"=w523:dbl[], "EPR_발생_total"=w529:i16[], "ERP_all"=w517:dbl[][], "ERP_Parameters"=w526:dbl[][])  [unwired: 2 in]
                n187 = Transpose 2D Array(2D array=w517) -> (transposed array=w516:dbl[][])
                n188 = Build Array (concatenate)(w527, w529) -> (w528:i16[])
                n189 = Build Array (concatenate)(w524, w526) -> (w525:dbl[][])
                n190 = Build Array (concatenate)(w514, w516) -> (w515:dbl[][])
                n191 = Build Array (concatenate)(w521, w523) -> (w522:dbl[])
                n192 = Build Array (concatenate)(w518, w520) -> (w519:dbl[])
                n193 = Build Array (concatenate)(w531, w532) -> (w530:i32[])
                n194 = Build Array (concatenate)(w536, w535) -> (w534:i32[][])
                n195 = global read "Control_Panel_정리.vi" "Target_Command"() -> (w506:i32)
                n196 = Equal?(x=w505, y=w532) -> (x = y?=w542:bool)
                n197 = Boolean To (0,1)(Boolean=w542) -> (0, 1=w539:i16)
                n198 = Build Array (concatenate)(w541, w505) -> (w540:i32[])
                n199 = Build Array (concatenate)(w538, w539) -> (w537:i16[])
                n200 = Equal?(x=w506, y=w505) -> ()  [unwired: 1 out]
              }
              frame #3 {
                # "0 = 온도\n1 = 자판\n2 = 침대\n3 = 용변 \n4 = 기계 \n5 = 응급"
                n201 = disable-structure shown="활성화" {
                  disable-tunnel: w558 -> [w576 w679]
                  disable-tunnel: w557 -> [w575 w678]
                  disable-tunnel: w556 -> [w574 _]
                  disable-tunnel: w555 -> [w573 _]
                  disable-tunnel: [w572 _] -> w554
                  disable-tunnel: [w571 _] -> w553
                  frame Enabled {
                    n202 = flat-sequence {
                      tunnel: w576 -> [w583]
                      tunnel: w575 -> [w577]
                      tunnel: w574 -> [w582]
                      tunnel: w573 -> [w581]
                      tunnel: [w580] -> w570
                      tunnel: [w579] -> w569
                      tunnel: [w668] -> w571
                      tunnel: [w669] -> w572
                      tunnel: w570 -> [w669]
                      tunnel: w569 -> [w668]
                      frame #0 {
                        n203 = case shown="참" w577 {
                          tunnel: w583 -> [_ w592]
                          tunnel: ["No Decesion" ("메시지") w591] -> w578
                          tunnel: w582 -> [w584 w590]
                          tunnel: w581 -> [w585 w589]
                          tunnel: [w585 w588] -> w580
                          tunnel: [w584 w587] -> w579
                          frame False {
                          }
                          frame True {
                            n204 = disable-structure shown="Enabled" {
                              disable-tunnel: [w598 _ "" ("메시지")] -> w591
                              disable-tunnel: w592 -> [w597 w640 _]
                              disable-tunnel: w590 -> [w596 _ _]
                              disable-tunnel: w589 -> [w595 _ _]
                              disable-tunnel: [w594 _ _] -> w588
                              disable-tunnel: [w593 _ _] -> w587
                              frame Enabled {
                                n205 = case shown="0" w597 {
                                tunnel: ["전원" ("메시지") "음향 UP" ("메시지") "채널 UP" ("메시지") "전체종료" ("메시지") "음향 Down" ("메시지") "채널 Down" ("메시지") "No Decesion" ("메시지")] -> w598
                                tunnel: w596 -> [w602 w609 w615 w620 w626 w633 w637]
                                tunnel: w595 -> [w601 w608 w616 w621 w625 w632 w638]
                                tunnel: [w600 w607 w614 w621 w624 w631 w638] -> w594
                                tunnel: [w599 w606 w613 w620 w623 w630 w637] -> w593
                                frame 0 {
                                n206 = VISA Write(VISA resource name=w601, write buffer="0", error in (no error)=w602) -> (VISA resource name out=w600:refnum<visa-resource-name>, error out=w599:errorcluster)  [unwired: 1 out]
                                n207 = Wait (ms)(milliseconds to wait=u32 10) -> ()  [unwired: 1 out]
                                }
                                frame 1 {
                                n208 = VISA Write(VISA resource name=w608, write buffer="L", error in (no error)=w609) -> (VISA resource name out=w607:refnum<visa-resource-name>, error out=w606:errorcluster)  [unwired: 1 out]
                                n209 = Wait (ms)(milliseconds to wait=u32 10) -> ()  [unwired: 1 out]
                                }
                                frame 2 {
                                n210 = VISA Write(VISA resource name=w616, write buffer="J", error in (no error)=w615) -> (VISA resource name out=w614:refnum<visa-resource-name>, error out=w613:errorcluster)  [unwired: 1 out]
                                n211 = Wait (ms)(milliseconds to wait=u32 10) -> ()  [unwired: 1 out]
                                }
                                frame 3 {
                                }
                                frame 4 {
                                n212 = VISA Write(VISA resource name=w625, write buffer="M", error in (no error)=w626) -> (VISA resource name out=w624:refnum<visa-resource-name>, error out=w623:errorcluster)  [unwired: 1 out]
                                n213 = Wait (ms)(milliseconds to wait=u32 10) -> ()  [unwired: 1 out]
                                }
                                frame 5 {
                                n214 = VISA Write(VISA resource name=w632, write buffer="K", error in (no error)=w633) -> (VISA resource name out=w631:refnum<visa-resource-name>, error out=w630:errorcluster)  [unwired: 1 out]
                                n215 = Wait (ms)(milliseconds to wait=u32 10) -> ()  [unwired: 1 out]
                                }
                                frame 9, Default {
                                }
                                }
                              }
                              frame Disabled {
                                n216 = case shown="0, 기본" w640 {
                                frame 0, Default {
                                n217 = Current VI's Path() -> (path=w642:path)
                                n218 = Strip Path(path=w642) -> (stripped path=w643:path)  [unwired: 1 out]
                                n219 = Build Path(base path=w643, name or relative path="0.wav" ("이름 또는 상대 경로")) -> (appended path=w641:path)
                                n220 = call "Sound_Sub.vi"("path"=w641) -> ()
                                }
                                frame 2 {
                                n221 = Current VI's Path() -> (path=w645:path)
                                n222 = Strip Path(path=w645) -> (stripped path=w646:path)  [unwired: 1 out]
                                n223 = Build Path(base path=w646, name or relative path="2.wav" ("이름 또는 상대 경로")) -> (appended path=w648:path)
                                n224 = call "Sound_Sub.vi"("path"=w648) -> ()
                                }
                                frame 3 {
                                n225 = Current VI's Path() -> (path=w649:path)
                                n226 = Strip Path(path=w649) -> (stripped path=w650:path)  [unwired: 1 out]
                                n227 = Build Path(base path=w650, name or relative path="3.wav" ("이름 또는 상대 경로")) -> (appended path=w652:path)
                                n228 = call "Sound_Sub.vi"("path"=w652) -> ()
                                }
                                frame 4 {
                                n229 = Current VI's Path() -> (path=w653:path)
                                n230 = Strip Path(path=w653) -> (stripped path=w654:path)  [unwired: 1 out]
                                n231 = Build Path(base path=w654, name or relative path="4.wav" ("이름 또는 상대 경로")) -> (appended path=w656:path)
                                n232 = call "Sound_Sub.vi"("path"=w656) -> ()
                                }
                                frame 5 {
                                n233 = Current VI's Path() -> (path=w657:path)
                                n234 = Strip Path(path=w657) -> (stripped path=w658:path)  [unwired: 1 out]
                                n235 = Build Path(base path=w658, name or relative path="5.wav" ("이름 또는 상대 경로")) -> (appended path=w660:path)
                                n236 = call "Sound_Sub.vi"("path"=w660) -> ()
                                }
                                frame 1 {
                                n237 = Current VI's Path() -> (path=w662:path)
                                n238 = Strip Path(path=w662) -> (stripped path=w663:path)  [unwired: 1 out]
                                n239 = Build Path(base path=w663, name or relative path="1.wav" ("이름 또는 상대 경로")) -> (appended path=w661:path)
                                n240 = call "Sound_Sub.vi"("path"=w661) -> ()
                                }
                                }
                              }
                              frame Disabled {
                              }
                            }
                          }
                        }
                        n241 = global write "Control_Panel_정리.vi" "선택된 기능"(w578) -> ()
                      }
                      frame #1 {
                        n242 = global read "Control_Panel_정리.vi" "Send_Interaction"() -> (w666:u8)
                        n243 = stacked-sequence {
                          tunnel: w666 -> [w671 _ w676]
                          tunnel: u32 0 ("dwFlags") -> [w670 _ w675]
                          frame #0 {
                            n244 = dll-call lib="User32.dll" fn="keybd_event"("bVk"=w671, "bScan"=w670, "dwFlags"=w670, "dwExtraInfo"=w670) -> ()  [unwired: 8 in, 2 out]
                          }
                          frame #1 {
                            n245 = global write "Control_Panel_정리.vi" "Switch"(FALSE ("Switch")) -> ()
                            n246 = Wait Until Next ms Multiple(millisecond multiple=u32 250) -> ()  [unwired: 1 out]
                          }
                          frame #2 {
                            n247 = dll-call lib="User32.dll" fn="keybd_event"("bVk"=w676, "bScan"=w675, "dwFlags"=u32 2, "dwExtraInfo"=w675) -> ()  [unwired: 8 in, 2 out]
                          }
                        }
                      }
                    }
                  }
                  frame Disabled {
                    n248 = case shown="참" w678 {
                      tunnel: w679 -> [_ w682]
                      tunnel: ["No Decesion" ("메시지") w681] -> w677
                      frame False {
                      }
                      frame True {
                        n249 = disable-structure shown="활성화" {
                          disable-tunnel: [w684 _ "" ("메시지")] -> w681
                          disable-tunnel: w682 -> [w683 w692 _]
                          frame Enabled {
                            n250 = case shown="5" w683 {
                              tunnel: ["온도" ("메시지") "자판" ("메시지") "침대" ("메시지") "용변" ("메시지") "기계" ("메시지") "응급" ("메시지") "No Decesion" ("메시지")] -> w684
                              frame 0 {
                              }
                              frame 1 {
                              }
                              frame 2 {
                              }
                              frame 3 {
                              }
                              frame 4 {
                              }
                              frame 5 {
                              }
                              frame 9, Default {
                              }
                            }
                          }
                          frame Disabled {
                            n251 = case shown="4" w692 {
                              frame 0, Default {
                                n252 = Current VI's Path() -> (path=w694:path)
                                n253 = Strip Path(path=w694) -> (stripped path=w695:path)  [unwired: 1 out]
                                n254 = Build Path(base path=w695, name or relative path="0.wav" ("이름 또는 상대 경로")) -> (appended path=w693:path)
                                n255 = call "Sound_Sub.vi"("path"=w693) -> ()
                              }
                              frame 2 {
                                n256 = Current VI's Path() -> (path=w697:path)
                                n257 = Strip Path(path=w697) -> (stripped path=w698:path)  [unwired: 1 out]
                                n258 = Build Path(base path=w698, name or relative path="2.wav" ("이름 또는 상대 경로")) -> (appended path=w700:path)
                                n259 = call "Sound_Sub.vi"("path"=w700) -> ()
                              }
                              frame 3 {
                                n260 = Current VI's Path() -> (path=w701:path)
                                n261 = Strip Path(path=w701) -> (stripped path=w702:path)  [unwired: 1 out]
                                n262 = Build Path(base path=w702, name or relative path="3.wav" ("이름 또는 상대 경로")) -> (appended path=w704:path)
                                n263 = call "Sound_Sub.vi"("path"=w704) -> ()
                              }
                              frame 4 {
                                n264 = Current VI's Path() -> (path=w705:path)
                                n265 = Strip Path(path=w705) -> (stripped path=w706:path)  [unwired: 1 out]
                                n266 = Build Path(base path=w706, name or relative path="4.wav" ("이름 또는 상대 경로")) -> (appended path=w708:path)
                                n267 = call "Sound_Sub.vi"("path"=w708) -> ()
                              }
                              frame 5 {
                                n268 = Current VI's Path() -> (path=w709:path)
                                n269 = Strip Path(path=w709) -> (stripped path=w710:path)  [unwired: 1 out]
                                n270 = Build Path(base path=w710, name or relative path="5.wav" ("이름 또는 상대 경로")) -> (appended path=w712:path)
                                n271 = call "Sound_Sub.vi"("path"=w712) -> ()
                              }
                              frame 1 {
                                n272 = Current VI's Path() -> (path=w714:path)
                                n273 = Strip Path(path=w714) -> (stripped path=w715:path)  [unwired: 1 out]
                                n274 = Build Path(base path=w715, name or relative path="1.wav" ("이름 또는 상대 경로")) -> (appended path=w713:path)
                                n275 = call "Sound_Sub.vi"("path"=w713) -> ()
                              }
                            }
                          }
                          frame Disabled {
                          }
                        }
                      }
                    }
                    n276 = global write "Control_Panel_정리.vi" "선택된 기능"(w677) -> ()
                  }
                }
              }
            }
            n277 = Increment(x=w139) -> (x+1=w138:i32)
            n278 = Build Array (concatenate)(w148, w147) -> (w141:dbl[])
          }
        }
        n279 = global read "Control_Panel_정리.vi" "정지"() -> (w88:bool)
      }
      n280 = global write "Control_Panel_정리.vi" "Acquisition Mode"(TRUE ("Device Control Enabled")) -> ()
      n281 = global write "Control_Panel_정리.vi" "Device Control Enabled"(FALSE ("Device Control Enabled")) -> ()
    }
    frame #3 {
      n282 = VISA Close(VISA resource name=w720, error in (no error)=w719) -> ()  [unwired: 1 out]
      n283 = dll-call lib="C:/Users/Server/Desktop/NeuroSky/NeuroSky_Dll_Call/Debug/NeuroSky_Dll_Call.dll" fn="FreeConnection"() -> ()  [unwired: 4 in, 2 out]
      n284 = global write "Control_Panel_정리.vi" "Acquisition Mode"(FALSE ("Device Control Enabled")) -> ()
      n285 = global write "Control_Panel_정리.vi" "Communication Stopped"(TRUE ("Device Control Enabled")) -> ()
      n286 = Build Path(base path=w723, name or relative path="Brain.txt") -> (appended path=w762:path)
      n287 = Build Path(base path=w723, name or relative path="selectedtarget.txt") -> (appended path=w754:path)
      n288 = Build Path(base path=w723, name or relative path="mius_flash_order.txt") -> (appended path=w759:path)
      n289 = Build Path(base path=w723, name or relative path="Target_order.txt") -> (appended path=w749:path)
      n290 = Build Path(base path=w723, name or relative path="Accuracy.txt") -> (appended path=w752:path)
      n291 = Build Path(base path=w723, name or relative path="ERP_발생_total.txt") -> (appended path=w742:path)
      n292 = Build Path(base path=w723, name or relative path="ERP_all_icon.txt") -> (appended path=w738:path)
      n293 = Build Path(base path=w723, name or relative path="ERP_total.txt") -> (appended path=w726:path)
      n294 = Build Path(base path=w723, name or relative path="SWLDA_hyperplane_value.txt") -> (appended path=w734:path)
      n295 = Build Path(base path=w723, name or relative path="decision_value.txt") -> (appended path=w731:path)
      n296 = call-poly <vilib>:"Write To Spreadsheet File.vi"("format (%.3f)"="%.6f", "1D data"=w718, "file path (dialog if empty)"=w762) -> ()  [unwired: 5 in, 1 out]
      n297 = call-poly <vilib>:"Write To Spreadsheet File.vi"("1D data"=w753, "file path (dialog if empty)"=w754) -> ()  [unwired: 6 in, 1 out]
      n298 = call-poly <vilib>:"Write To Spreadsheet File.vi"("transpose? (no:F)"=TRUE, "2D data"=w757, "file path (dialog if empty)"=w759) -> ()  [unwired: 5 in, 1 out]
      n299 = call-poly <vilib>:"Write To Spreadsheet File.vi"("transpose? (no:F)"=TRUE, "1D data"=w746, "file path (dialog if empty)"=w749) -> ()  [unwired: 5 in, 1 out]
      n300 = call-poly <vilib>:"Write To Spreadsheet File.vi"("1D data"=w750, "file path (dialog if empty)"=w752) -> ()  [unwired: 6 in, 1 out]
      n301 = call-poly <vilib>:"Write To Spreadsheet File.vi"("transpose? (no:F)"=TRUE, "1D data"=w740, "file path (dialog if empty)"=w742) -> ()  [unwired: 5 in, 1 out]
      n302 = call-poly <vilib>:"Write To Spreadsheet File.vi"("transpose? (no:F)"=TRUE, "format (%.3f)"="%.6f", "2D data"=w735, "file path (dialog if empty)"=w738) -> ()  [unwired: 4 in, 1 out]
      n303 = call-poly <vilib>:"Write To Spreadsheet File.vi"("transpose? (no:F)"=TRUE, "format (%.3f)"="%.6f", "2D data"=w724, "file path (dialog if empty)"=w726) -> ()  [unwired: 4 in, 1 out]
      n304 = call-poly <vilib>:"Write To Spreadsheet File.vi"("format (%.3f)"="%.6f", "1D data"=w732, "file path (dialog if empty)"=w734) -> ()  [unwired: 5 in, 1 out]
      n305 = call-poly <vilib>:"Write To Spreadsheet File.vi"("format (%.3f)"="%.6f", "1D data"=w729, "file path (dialog if empty)"=w731) -> ()  [unwired: 5 in, 1 out]
    }
    frame #4 {
      n306 = global write "Control_Panel_정리.vi" "Communication Stopped"(FALSE ("Device Control Enabled")) -> ()
    }
  }
